vi "PopTop.vi"(0 "Message":string) -> ()   [LabVIEW 2014]
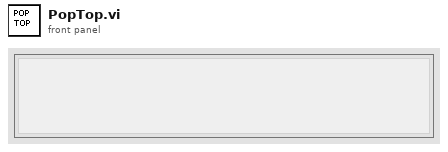
[diagram p1: front panel]
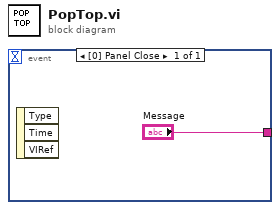
[diagram p0: block diagram]
diagram:
  n1 = event shown="[0] Panel Close" {
    selector: _ -> [_]
    dyn-events: _ -> [_]
    timeout: _ -> [_]
    tunnel: ["Message"] -> _
    event Panel Close {
      n2 = event-data() -> ()  [unwired: 1 in, 3 out]
    }
  }
